vi "Restore General Property.vi"(4 "Control Ref Cluster":T1, 6 "Update?":bool=TRUE, 8 "error in (no error)":errorcluster, 11 "2D Plot.lvclass in":refnum<class "2D Plot.lvclass">) -> (0 "error out":errorcluster, 3 "2D Plot.lvclass out":refnum<class "2D Plot.lvclass">)   [LabVIEW 2017, in "2D Plot.lvclass"]
uses:
  <vilib>/Math Plots/2D Math Plots/2D Plot/2D Plot/2D Plot.lvclass
  <vilib>/Math Plots/2D Math Plots/2D Plot/Action String/2DMathPlot Ctrl Act Cluster.ctl
  <vilib>/Math Plots/2D Math Plots/2D Plot/Action String/2DMathPlot State Class.ctl
  <vilib>/Math Plots/2D Math Plots/2D Plot/2D Plot/2D Plot.lvclass/2D Plot.ctl
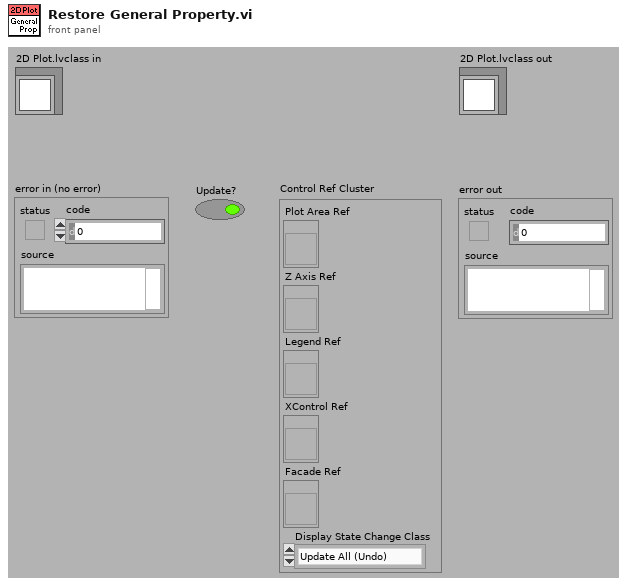
[diagram p1: front panel]
types:
  T1 = typedef "2DMathPlot Ctrl Act Cluster.ctl" = cluster{"Plot Area Ref":refnum<vi>, "Z Axis Ref":refnum<vi>, "Legend Ref":refnum<vi>, "XControl Ref":refnum<vi>, "Facade Ref":refnum<vi>, "Display State Change Class":T2}
  T2 = typedef "2DMathPlot State Class.ctl" = enum16{"Update All (Undo)", "Update General", "Update Appearance", "Update Format", "Update Scale", "Update Marker", "Update Cursor", "None"}
  T3 = typedef "LVAnnotationListTypeDef.ctl" = cluster{"Name":string, "Color":u32, "Style":u8, "Point Style":u8, "Name Visible":bool, "Allow Drag":bool, "Annotation Mode":u32, "Plot":i32, "Index":i32, "Position":cluster{"X":dbl, "Y":dbl}, "X Scale":u32, "Y Scale":u32, "Show Arrow":bool, "Lock Name":bool, "Plot Area":i32, "Label Offset":cluster{"X":dbl, "Y":dbl}}[]
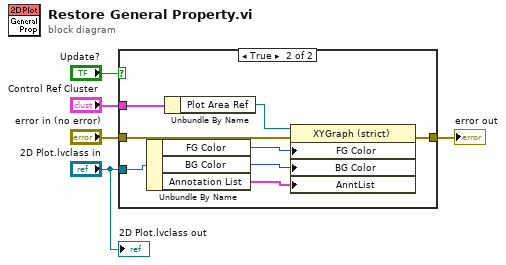
[diagram p0: block diagram]
diagram:
  n1 = case shown="True" "Update?" {
    tunnel: "2D Plot.lvclass in" -> [_ w14]
    tunnel: "Control Ref Cluster" -> [_ w9]
    tunnel: "error in (no error)" -> [w6 w8]
    tunnel: [w6 w7] -> w3
    frame False {
    }
    frame True {
      n2 = Unbundle By Name(w14) -> ("FG Color"=w13:u32, "BG Color"=w12:u32, "Annotation List"=w11:T3)
      n3 = Unbundle By Name(w9) -> ("Plot Area Ref"=w10:refnum<vi>)
      n4 = property class="XYGraph (strict)"(reference=w10, error in=w8, "FG Color"=w13, "BG Color"=w12, "AnntList"=w11) -> (error out=w7:errorcluster)  [unwired: 1 out]
    }
  }
  "error out" <- w3
  "2D Plot.lvclass out" <- "2D Plot.lvclass in"
